vi "AlliGator Load Dataset or Series.vi"(4 "Save Phasor Plot with Overlay":bool, 6 "Save Image with Overlay":bool, 7 "VI in":refnum<vi>, 8 "error in (no error)":errorcluster, 9 "Type of Displayed Image":T1 caption="Displayed Image", 10 "File/Folder Path":path, 11 "AlliGator Ctrl Refnums":T2) -> (0 "error out":errorcluster, 1 "Message":string, 3 "AlliGator Q Elements out":T11[](array[typedef]))   [LabVIEW 2021, in "AlliGator Files.lvlib"]
doc: "Detects type of file loaded and generates the series of actions needed to load it."
uses:
  AlliGator Files.lvlib
  Action Engine/AlliGator Q Element.ctl
  Action Engine/AlliGator Q Event.ctl
  GUI/AlliGator Ctrl Refnums.ctl
  GUI/AlliGator Other Ctrl Refnums.ctl
  GUI/AlliGator State Indicator.ctl
  GUI/AlliGator Main Window Tabs.ctl
  GUI/AlliGator Phasor Plot Ctrl Refnums.ctl
  GUI/AlliGator Phasor Graph Ctrl Refnums.ctl
  Phasor/Phasor Calibration Type.ctl
  GUI/AlliGator Dataset Ctrl Refnums.ctl
  Source Image/AlliGator Displayed Image.ctl
  GUI/AlliGator Registered Events Ctrl Refnums.ctl
  GUI/AlliGator Image Histogram Control Refnums.ctl
  Histograms/Linear Histogram Options.ctl
  Histograms/Histogram Bin Option.ctl
  Histograms/Histogram Bin Position.ctl
  Decay Fit Parameter Map/AlliGator Decay Fit Map Control Refnums.ctl
  Fits/IRF(X)PSED/Decay Fit Parameters & Derived Quantities List v2.ctl
  Parameter Map/AlliGator Parameter Map Control Refnums.ctl
  Files/Load-Save File Info.ctl
  AlliGator FLI Dataset Type.ctl
  ROIs/AlliGator ROI Manager Actions.ctl
  AlliGator Select Folder Mode.ctl
  AlliGator Folder Selection.ctl
  <vilib>/Utility/error.llb/Error Cluster From Error Code.vi
  ROIs/AlliGator Source Image ROI Storage [SGL] v3.vi
  <userlib>/_OpenG.lib/array/array.llb/Filter 1D Array with Scalar (String)__ogtk.vi
  <vilib>/ErrorRing/Error Ring.xnode
  HDF5/AlliGator HDF5.lvlib
  <userlib>/_OpenG.lib/file/file.llb/openg_file.lvlib
  Files/Files.lvlib
  Image/Image.lvlib
  Action Engine/AlliGator Action Engine.lvlib
  <userlib>/_OpenG.lib/array/array.llb/openg_array.lvlib
  ROIs/AlliGator ROIs.lvlib
  Graphs/XY Graph/XY Graph Add-Ons.lvlib
  Globals, Variables, Constants/AlliGator Globals, Variables & Constants.lvlib
  Scripts/AlliGator Scripts.lvlib
  Decay Fit Parameter Map/AlliGator Decay Fit Parameter Map.lvlib
  GUI/GUI.lvlib
  Settings/AlliGator Settings.lvlib
  Sound/Sound.lvlib
  Source Image/AlliGator Source Image.lvlib
  GUI/AlliGator GUI.lvlib
  Phasor/Phasor.lvlib
  Histograms/Histogram Window.lvlib
  Fits/Fits.lvlib
  Parameter Map/AlliGator Parameter Map.lvlib
panel:
  out "Script out":bool
  in  "Script in":bool
  # "see the AlliGator License on the block diagram (Ctrl+E or Window:Show Block Diagram)"
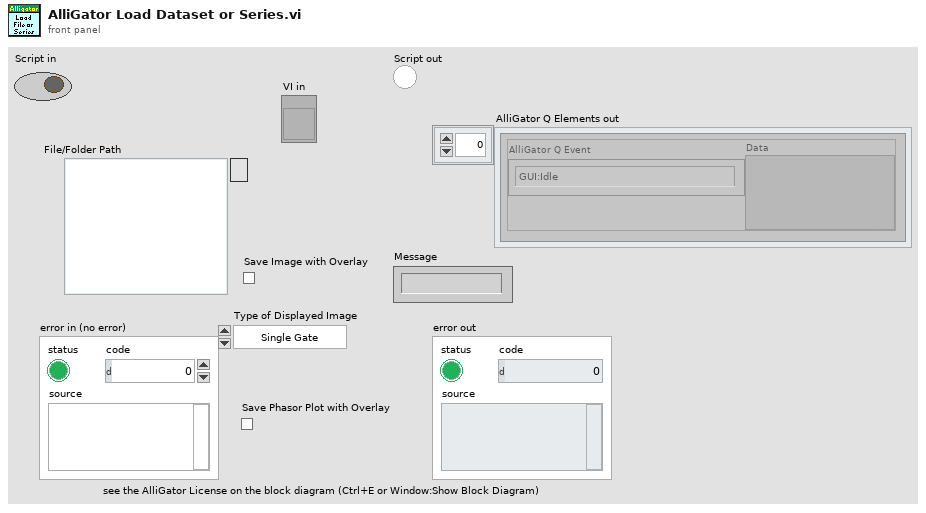
[diagram p1: front panel]
types:
  T1 = typedef "AlliGator Source Image.lvlib/AlliGator Displayed Image.ctl" = enum16{"Single Gate", "Sum of All Gates", "Max of All Gates", "Min of All Gates", "-", "White Ligth Image", "Mask Image"}
  T2 = typedef "AlliGator GUI.lvlib/AlliGator Ctrl Refnums.ctl" = cluster{"Other AlliGator Ctrl Refnums":T3, "Phasor Plot Ctrl Refnums":T4, "Phasor Graph Ctrl Refnums":T5, "Dataset Control References":T6, "Registered Events Ctrl Refnums":T7, "Image Histogram Ctrl Refnums":T8, "Decay Fit Map Ctrl Refums":T9, "Parameter Map Ctrl Refums":T10}
  T3 = typedef "AlliGator GUI.lvlib/AlliGator Other Ctrl Refnums.ctl" = cluster{"State Indicators":refnum<vi>, " Progress Bar":refnum<vi>, "Decay Graph Active":refnum<vi>, "Decay Statistics Bin":refnum<vi>, "Time Step":refnum<vi>, "Use File Timestamp":refnum<vi>, "Tab Control":refnum<vi>, "CPU":refnum<vi>, "Abort Fit":refnum<vi>, "Dataset File/Folder Path":refnum<vi>, "Abort ROI Creation":refnum<vi>, "Event LED":refnum<vi>, "Dataset File/Folder Path 2":refnum<vi>, "Dataset File/Folder Path 3":refnum<vi>, "Dataset File/Folder Path 4":refnum<vi>, "Dataset File/Folder Path 5":refnum<vi>, "Dataset File/Folder Path 6":refnum<vi>, "Dataset File/Folder Path 7":refnum<vi>, "Dataset File/Folder Path 8":refnum<vi>, "Dataset File/Folder Path 9":refnum<vi>, "Dataset File/Folder Path 10":refnum<vi>, "Dataset File/Folder Path 11":refnum<vi>}
  T4 = typedef "AlliGator GUI.lvlib/AlliGator Phasor Plot Ctrl Refnums.ctl" = cluster{"Phasor Ratio":refnum<vi>, "Modulus Lifetime":refnum<vi>, "Phasor at cursor (m, phi)":refnum<vi>, "Phase Lifetime":refnum<vi>, "Phasor at cursor (g, s)":refnum<vi>, "Phasor Plor Average Lifetime":refnum<vi>, "Phasor Plot Active":refnum<vi>, "Save Phasor Plot":refnum<vi>, "Image Overlay Color":refnum<vi>, "Phasor Plot Color Scale":refnum<vi>, "Reference 1 Button":refnum<vi>, "Reference 2 Button":refnum<vi>}
  T5 = typedef "AlliGator GUI.lvlib/AlliGator Phasor Graph Ctrl Refnums.ctl" = cluster{"Phasor Ratio":refnum<vi>, "Modulus Lifetime":refnum<vi>, "Phasor at cursor (m, phi)":refnum<vi>, "Phase Lifetime":refnum<vi>, "Phasor at cursor (g, s)":refnum<vi>, "Phasor Graph Average Lifetime":refnum<vi>, "Phasor Graph Active":refnum<vi>, "Save Phasor Graph":refnum<vi>, "Phasor Frame Slide":refnum<vi>, "Single Step Phasor":refnum<vi>, "Calibration Type":refnum<vi>, "Show Line":refnum<vi>, "Phase Lifetime 1":refnum<vi>, "Phase Lifetime 2":refnum<vi>, "Phasor Graph Frequency":refnum<vi>, "Phasor Reference 1 Control":refnum<vi>, "Phasor Reference 2 Control":refnum<vi>, "Calibration Lifetime":refnum<vi>, "Phase Lifetime SDV":refnum<vi>, "Average Lifetime SDV":refnum<vi>, "Phasor Ratio SDV":refnum<vi>, "Modulus Lifetime SDV":refnum<vi>}
  T6 = typedef "AlliGator GUI.lvlib/AlliGator Dataset Ctrl Refnums.ctl" = cluster{"Current Data":refnum<vi>, "Gate Image Slide":refnum<vi>, "Time Point Slide":refnum<vi>, "Current Time Stamp":refnum<vi>, "Save Image":refnum<vi>, "Displayed Image":refnum<vi>, "Overlay Mode":refnum<vi>, "Phasor Overlay Color":refnum<vi>, "Image Color Scale":refnum<vi>, "Use ROI as Search Area":refnum<vi>, "Source Image ROI Color":refnum<vi>}
  T7 = typedef "AlliGator GUI.lvlib/AlliGator Registered Events Ctrl Refnums.ctl" = cluster{"Time Point Slider":refnum<vi>, "Phasor Plot Display Range":refnum<vi>, "Decay Graph":refnum<vi>, "Decay Statistics Graph":refnum<vi>, "Intensity Time Trace":refnum<vi>, "Phasor Graph":refnum<vi>, "Phasor Ratio Graph":refnum<vi>, "Lifetime Graph":refnum<vi>, "Phasor Plot Display":refnum<vi>, "Source Image Display":refnum<vi>, "Decay Fit Parameter Map Display Range":refnum<vi>, "Decay Fit Parameter Map Display":refnum<vi>, "Parameter Map Display Range":refnum<vi>, "Parameter Map Display":refnum<vi>, "Phasor Plot Display Range":refnum<vi>}
  T8 = typedef "AlliGator GUI.lvlib/AlliGator Image Histogram Control Refnums.ctl" = cluster{"Image Histogram":refnum<vi>, "Image Histogram Options":refnum<vi>, "Image Histogram Active":refnum<vi>, "Image Histogram Upper Percentile":refnum<vi>, "Image Histogram Lower Percentile":refnum<vi>, "Auto-Adjust Contrast":refnum<vi>}
  T9 = typedef "AlliGator Decay Fit Parameter Map.lvlib/AlliGator Decay Fit Map Control Refnums.ctl" = cluster{"Decay Fit Parameter Map Color Scale":refnum<vi>, "Decay Fit Parameter":refnum<vi>, "Max Parameter":refnum<vi>, "Min Parameter":refnum<vi>, "Decay Fit Parameter Map Display":refnum<vi>, "Decay Fit Parameter Map Display Range":refnum<vi>}
  T10 = typedef "AlliGator Parameter Map.lvlib/AlliGator Parameter Map Control Refnums.ctl" = cluster{"Parameter Map Color Scale":refnum<vi>, "Map Parameter":refnum<vi>, "Max Parameter":refnum<vi>, "Min Parameter":refnum<vi>, "Parameter Map Display":refnum<vi>, "Parameter Map Display Range":refnum<vi>, "Parameter Map Set":refnum<vi>}
  T11 = typedef "AlliGator Action Engine.lvlib/AlliGator Q Element.ctl" = cluster{"AlliGator Q Event":T12, "Data":variant}
  T12 = typedef "AlliGator Action Engine.lvlib/AlliGator Q Event.ctl" = enum16{"---- Files ----", "Files:Set Batch Export Files To Save", "Files:Set Dataset Loading & Pre-processing Options", "Files:Check #Frames in Dataset", "Files:Increment Frame Index", "Files:Open Mask Image", "Files:Open White Light Image", "Files:Open Single Dataset", "Files:New Folder of Folders Selected", "Files:Load File (all Types)_Scriptable", "Files:Move Flattened Series to Folders Series", "Files:Select Folder", "Files:Load FLI Dataset", "Files:Load Swiss SPAD 1 Dataset", "Files:Load Swiss SPAD 2 Dataset", "Files:Load .sdt FLI Dataset", "Files:Load .ptu FLI Dataset", "Files:Load .bin FLI Dataset", "Files:Load Single Gate Image Folder", "Files:Load I/m/phi Dataset (deprecated)", "Files:Load Single Image", "Files:Subtract Background File", "Files:Export FLI Dataset", "Files:Load HDF5 FLI Dataset", "Files:Set Destination File Path", "Files:Save Mask Image", "Files:Batch Conversion", "Files:New Folder Selected", "Files:Close FLI Dataset", "Files:Close FLI Dataset Series", "Files:Close White Light Image", "Files:Close Mask Image", "---- FLI Dataset ----", "FLI Dataset:Channel Arithmetic", "FLI Dataset:Export Average Lifetime Map as ASCII", "FLI Dataset:Export User-Defined Quantity Map as ASCII", "FLI Dataset:Python Function FLI Dataset Event", "FLI Dataset:ROI Analysis", "FLI Dataset:Tilted Logistic Square Gated IRF Characteristics Map", "FLI Dataset:Logistic Square Gated IRF Characteristics Map", "FLI Dataset:Square Gated IRF Characteristics Map", "FLI Dataset:Multi-ROI Single-Pixel Phasor Analysis", "FLI Dataset:Multi-ROI Single-Pixel NLSF Analysis", "FLI Dataset:All ROIs IRF Extraction", "FLI Dataset:All ROIs Decay Fit Non-Interactive (Fast + Individual IRF)", "FLI Dataset:All ROIs Phasor Analysis", "FLI Dataset:All ROIs Decay Fit", "FLI Dataset:Fluorescence Decay Statistics", "FLI Dataset:Update Decay Statistics Graph", "FLI Dataset:Get Decay from ROI", "FLI Dataset:All ROIs Average Lifetimes", "FLI Dataset:Save/Load Local IRFs", "FLI Dataset:Clear Local IRFs", "---- FLI Dataset Series ----", "FLI Dataset Series:Sum All Datasets in Series", "FLI Dataset Series:Add Dataset to Accumulated Dataset", "FLI Dataset Series:Display Accumulated Dataset", "FLI Dataset Series:Clear Dataset Series Sum", "FLI Dataset Series:Time-Series Analysis (NLSF)", "FLI Dataset Series:Time-Series Analysis (Phasor)", "---- Image ----", "Image:Update Image Profile Plots", "Image:Image Histogram Cursor Move", "Image:Image Histogram", "Image:Image Contrast", "Image:Set Image Histogram Cursor Move Flag", "Image:Clear Image Overlay", "Image:Use ROI as Search Area", "Image:Set ROI Diameter", "Image:Save Image Data as TIFF", "Image:Save Displayed Image with Overlay", "Image:Save Image Overlay Only", "Image:Save Image as Hot Pixel Mask", "Image:Change Source Image Color Palette", "Image:Copy Image to Clipboard", "Image:Source Image ROI Selection", "Image:Delete All ROIs", "Image:Delete All Unselected ROIs", "Image:Delete ROI", "Image:Merge All ROIs", "Image:Store ROI", "Image:Source Image ROI Storage", "Image:Export ROI Description to Notebook", "Image:Save ROI", "Image:Load ROI", "Image:Paste ROI Definition", "Image:Clear ROI", "Image:Identify ROIs in Mask Image", "Image:Create Complementary ROI", "Image:Create Contour ROI", "Image:Create ROI(s) from Pixels with Peak above Min_Scriptable", "Image:Create ROI(s) from Pixels with Intensity above Min_Scriptable", "Image:Compute ROI Statistics", "Image:Delete ROI(s) based on ROI Characteristics", "Image:Create ROI Grid", "Image:ROI to Individual Pixel ROIs", "Image:Python Function Source Image Event", "Image:Show Phasor Calibration Map ROI Centers", "Image:Convert ROI to Mask Image", "Image:Mouse Move", "Image:Mouse Up", "Image:Set Source Image Mouse Move Flag", "Image:Add Scale Bar Overlay", "Image:Delete Existing ROIs Option", "Image:Overlay ROI Median", "Image:Check Current ROI", "---- Decay ----", "Decay:Clear IRF/Reference Plot", "Decay:Add Decay to Graph", "Decay:Smoothen Plot", "Decay:Smoothen Plot Tail", "Decay:Average Selected Plots", "Decay:Extract IRF", "Decay:Optimal IRF Extraction", "Decay:Threshold IRF", "Decay:Fit to Model IRF", "Decay:Fit IRF to Square Gate", "Decay:Fit IRF to Logistic Square Gate", "Decay:Fit IRF to Tilted Logistic Square Gate", "Decay:Create Bounding Cursors Set", "Decay:Export Bounding Cursors Definition to Notebook", "Decay:Denoise Plot", "Decay:Compute Cumulative Function", "Decay:Use as Reference Decay", "Decay:Show Reference Decay/IRF", "Decay:Extrapolate Decay", "Decay:Create Head & Tail Bounding Cursors", "Decay:Store Cursor-defined Head & Tail Fractions", "Decay:Rebin Plot", "Decay:1-Normalize Decay", "Decay:[0-1]-Normalize Plot", "Decay:Straighten Decay", "Decay:Shift Decay", "Decay:Fold Decay", "Decay:Fit Decay", "Decay:Global Fit of Selected Decays", "Decay:Post Global Fit Script", "Decay:Add Global Fit Parameters to Graph", "Decay:Add Decay Parameter(s) to Plot (Graph)", "Decay:Export Decay to Phasor Graph", "Decay:Plot Decay Shifts", "Decay:Compute Average Lifetime", "Decay:Plot Convolution", "Decay:Graph Tip Strip Update", "---- Decay Statistics ----", "Decay Statistics:Tip Strip Update", "---- Intensity Time Trace ----", "Intensity Time Trace:Use File Timestamp", "Intensity Time Trace:Load Intensity Corrections File", "Intensity Time Trace:Clear Intensity Corrections File", "Intensity Time Trace:Tip Strip Update", "---- Phasor Plot ----", "Phasor Plot:Build Phasor Plot", "Phasor Plot:Change Phasor Plot Color Palette", "Phasor Plot:Adjust Phasor Plot Display Range", "Phasor Plot:Highlight Image ROI in Phasor Plot", "Phasor Plot:Save Phasor Plot Image with Overlay", "Phasor Plot:Export Complex Phasor Map", "Phasor Plot:Export Phasor Ratio Map", "Phasor Plot:Export Average Lifetime Map", "Phasor Plot:Compute Phase Lifetime Histogram", "Phasor Plot:Compute Phasor Ratio Histogram", "Phasor Plot:Compute Phase Lifetime vs Intensity Scatter Plot", "Phasor Plot:Weber 2-Component Decomposition", "Phasor Plot:Update Phasor Color Map Vertices", "Phasor Plot:Clear Phasor Overlay", "Phasor Plot:Use Segment Extremities as References", "Phasor Plot:Use UC/Segment Intersections as References", "Phasor Plot:Use UC/Principal Axis Intersections as References", "Phasor Plot:Use UC/Linear Fit Intersections as References", "Phasor Plot:Update Phasor Plot Reference", "Phasor Plot:Show Local Phasor Info in Phasor Plot", "Phasor Plot:Update Phasor Plot State", "Phasor Plot:Phasor Plot ROI Storage", "Phasor Plot:Phasor Plot ROI Selection", "Phasor Plot:Python Function Phasor Plot Event", "Phasor Plot:Overlay Phasor ROI, Ratio or Map in Source Image", "Phasor Plot:Compute Decay of Selected Phasors", "Phasor Plot:Phasor at Image Pixel", "Phasor Plot:Mouse Move", "Phasor Plot:Mouse Up", "Phasor Plot:Display Range Mouse Move", "Phasor Plot:Set Mouse Move Flag", "---- Phasor Graph ----", "Phasor Graph:Calibrated Phasor Map Series", "Phasor Graph:Whole Image Phasor Scatter Plot (deprecated)", "Phasor Graph:Get Phasor Value", "Phasor Graph:Create New Phasor Plot Dialog", "Phasor Graph:Update Last Phasor Value", "Phasor Graph:Update Phasor (m, phi)", "Phasor Graph:Remove Single Phasor from Plot", "Phasor Graph:Add Single Phasor to Plot", "Phasor Graph:Remove Phasor Plot", "Phasor Graph:Remove Selected Phasor Plots", "Phasor Graph:Clear Phasor Data", "Phasor Graph:Clear Phasor Graph", "Phasor Graph:Cursor Move", "Phasor Graph:Draw Cursor Connecting Line", "Phasor Graph:Clear Cursor Connecting Line", "Phasor Graph:Find UC Intersection", "Phasor Graph:Use UC/Cursor-Defined Line Intersections", "Phasor Graph:Use Selected Plots Fitted Line/UC Intersections", "Phasor Graph:Use Selected Plots Principal Axis/UC Intersections", "Phasor Graph:Show Single Phasor", "Phasor Graph:Save Single Phasor Plot", "Phasor Graph:Save All Phasor Plots", "Phasor Graph:Load Phasor Plot(s)", "Phasor Graph:Phasor Multiplication", "Phasor Graph:Compute Average Phasor", "Phasor Graph:Compute Multiple Average Phasors (Selected Plots)", "Phasor Graph:Export Single Phasor Plot Phase Lifetimes", "Phasor Graph:Phase Lifetime Trajectory (deprecated)", "Phasor Graph:Phase Lifetime vs Intensity Scatter Plot (deprecated)", "Phasor Graph:Parameter 2 vs Parameter 1 Scatter Plot", "Phasor Graph:Use Cursor n Location", "Phasor Graph:Set Reference n to Current Phase Lifetime Value", "Phasor Graph:Set Reference n to Lifetime Value", "Phasor Graph:Set Cursor n Location", "Phasor Graph:Save Phasor Graph Image", "Phasor Graph:Update SEPL Plot", "Phasor Graph:Export Single Phasor Plot Data", "Phasor Graph:Export Selected Phasor Plots Data", "Phasor Graph:Python Function Phasor Graph Event", "Phasor Graph:Tip Strip Update", "---- Calibration ----", "Calibration:Set Calibration Type", "Calibration:Load/Save Phasor Calibration", "Calibration:Load/Save Phasor Calibration Series", "Calibration:Load/Save Phasor Calibration Map", "Calibration:Use as Calibration", "Calibration:Compute Optimal Calibration from Phasor References", "Calibration:Clear Phasor Calibration", "Calibration:Single Phasor Calibration Information", "Calibration:Use as Calibration Series", "Calibration:Use as Calibration Map", "Calibration:Clear Calibration Series", "Calibration:Phasor Calibration Series Information", "Calibration:Clear Calibration Map", "Calibration:Phasor Calibration Map Information", "Calibration:Apply Phasor Calibration", "Calibration:Update Single Plot Calibration", "Calibration:Update Multiple Plots Calibration", "Calibration:Clear Single Plot Calibration", "Calibration:Clear All Plots Calibrations", "Calibration:Clear Plot(s) Calibration(s)?", "Calibration:Phasor Calibration Maps (# Gates Series)", "---- Phasor Ratio ----", "Phasor Ratio:Clear Reference n", "Phasor Ratio:Toggle Selected Plot(s)  Lock to Reference 1", "Phasor Ratio:Use as Reference n", "Phasor Ratio:Send Reference n to Notebook", "Phasor Ratio:Toggle Selected Plot(s)  Lock to Reference 2", "Phasor Ratio:Compute Phasor Ratio at Mouse Location", "Phasor Ratio:Compute Phasor Plot's Average Phasor Ratio", "Phasor Ratio:Compute Time-Series Phasor Ratios", "Phasor Ratio:Fit Line to Phasor Ratio Plot", "Phasor Ratio:Save References", "Phasor Ratio:Load References", "Phasor Ratio:Update Phasor Reference 1", "Phasor Ratio:Update Phasor Reference 2", "Phasor Ratio:Move Cursor n to Reference n", "Phasor Ratio:Use as Phasor Reference 1 Lifetime", "Phasor Ratio:Use as Phasor Reference 2 Lifetime", "Phasor Ratio:Export Phasor Ratio Map as ASCII", "Phasor Ratio:Tip Strip Update", "---- Lifetime & Other Parameters Graph ----", "Lifetime:Power Law from Intensity Distribution", "---- Decay Fit Parameter Map ----", "Decay Fit Parameter Map:Export ROI NLSF Data as ASCII", "Decay Fit Parameter Map:Set Decay Fit Parameter Map Selection", "Decay Fit Parameter Map:Build Decay Fit Parameter Map", "Decay Fit Parameter Map:Change Decay Fit Parameter Map Color Palette", "Decay Fit Parameter Map:Export Decay Fit Parameter Map Data as ASCII", "Decay Fit Parameter Map:Export All Decay Fit Parameter Maps Data as ASCII", "Decay Fit Parameter Map:Selected Parameter Scatterplot", "Decay Fit Parameter Map:Parameter 2 vs Parameter 1 Scatterplot", "Decay Fit Parameter Map:Save Decay Fit Parameter Map Image", "Decay Fit Parameter Map:Save-Load IRFs & Fit Data", "Decay Fit Parameter Map:Update Local Decay Plots", "Decay Fit Parameter Map:Python Function Decay Fit Parameters Map Event", "Decay Fit Parameter Map:Overlay Decay Fit Parameter Map in Source Image", "Decay Fit Parameter Map:Selected Parameter vs Intensity Scatterplot", "Decay Fit Parameter Map:Mouse Up", "Decay Fit Parameter Map:Display Range Mouse Move", "---- Parameter Map ----", "Parameter Map:Export ROI Parameters Data as ASCII", "Parameter Map:Delete Parameter Map Set", "Parameter Map:Update Parameter List", "Parameter Map:Build Parameter Map", "Parameter Map:Change Parameter Map Color Palette", "Parameter Map:Export Parameter Map Data as ASCII", "Parameter Map:Export All Parameter Maps Data as ASCII", "Parameter Map:Selected Parameter Scatterplot", "Parameter Map:Parameter 2 vs Parameter 1 Scatterplot", "Parameter Map:Selected Parameter vs Intensity Scatterplot", "Parameter Map:Save Parameter Map Image", "Parameter Map:Save-Load IRFs & Parameter Maps (TODO)", "Parameter Map:Set Parameter Map Selection", "Parameter Map:Python Function Parameter Map Event", "Parameter Map:Overlay Parameter Map in Source Image", "Parameter Map:Update Local Decay Plots", "Parameter Map:Mouse Up", "Parameter Map:Display Range Mouse Move", "---- Generic Graph ----", "Generic Graph:Generic XY Graph Event", "Generic Graph:Python Function XY Graph Event", "Generic Graph:New Plot", "Generic Graph:Save Plot", "Generic Graph:XY Plot Histogram", "Generic Graph:Set XY Graph Plot Name", "Generic Graph:Set Last Cursor Style", "Generic Graph:Tip Strip Update", "---- GUI ----", "GUI:Start Script", "GUI:Type of Displayed Image Changed", "GUI:Gate Image Slide Changed", "GUI:Show Busy Icon", "GUI:Show Busy Icon & Abort Button", "GUI:Hide Busy Icon", "GUI:Hide Busy Icon & Abort Button", "GUI:Abort", "GUI:End Script", "GUI:Start Timing", "GUI:End Timing", "GUI:Set State Indicator", "GUI:Send Parameters JSON Strings to Clipboard", "GUI:Set Gate Step", "GUI:Idle", "GUI:Initialization", "GUI:Quit", "GUI:Increment Dataset Index", "GUI:Set Dataset Index to -1", "GUI:Time Series Slider Moved", "GUI:Time Series Slider Changed", "GUI:Toggle Playback or Loop", "GUI:Playback Script", "GUI:Set Phasor Frequency", "GUI:Open Window", "GUI:Start Test Script", "GUI:End Test Script", "DEBUG"}
  T13 = typedef "Files.lvlib/Load-Save File Info.ctl" = cluster{"Load/Save":bool, "File Path":path}
  T14 = typedef "AlliGator Files.lvlib/AlliGator FLI Dataset Type.ctl" = enum16{"HDF5 FLI Dataset", "Gate Image Folder", ".sdt FLI Dataset (Becker & Hickl)", ".ptu FLI Dataset (PicoQuant)", "SS1 FLI Dataset", "SS2 FLI Dataset", "I/m/phi Dataset", ".bin FLI Dataset (PicoQuant Binned)", ".bin FLI Dataset (Piccolo Binned)", ".mat FLI Dataset"}
  T15 = typedef "ROI Descriptor" = cluster{"Global Rectangle":i32[], "Contours":cluster{"ID":enum32{"External", "Internal"}, "Type":u32, "Coordinates":i32[]}[]}
  T16 = typedef "AlliGator ROIs.lvlib/AlliGator ROI Manager Actions.ctl" = enum16{"Undefined", "Delete Current ROI", "Delete All Unselected ROIs", "Delete Multiple ROIs", "Delete All ROIs", "Swap ROIs", "Insert ROI", "Update Current ROI Descriptor", "Rename Current ROI", "Store New ROI", "Store Multiple ROIs", "Select Next ROI", "Select Previous ROI", "Find Selected ROI", "Show All ROIs", "Update ROI Manager Window", "Merge All ROIs", "Unmerge ROI", "Set Selected ROI by ID"}
  T17 = typedef "AlliGator Files.lvlib/AlliGator Folder Selection.ctl" = cluster{"Folder Selection Mode":T18, "Folder Path":path}
  T18 = typedef "AlliGator Files.lvlib/AlliGator Select Folder Mode.ctl" = enum16{"Select Gate Folder", "Select Folder of Gate Folders", "Select Folder of SwissSPAD 2 Datasets", "Select Folder of .sdt FLI Datasets (Becker & Hickl)", "Select Folder of .ptu FLI Datasets (PicoQuant)", "Select Folder of .bin FLI Datasets (PicoQuant Binned)", "Select Folder of .bin FLI Datasets (Piccolo Binned)", "Select Folder of HDF5 FLI Datasets"}
  T19 = typedef "AlliGator HDF5 File Type.ctl" = enum16{"FLI Dataset", "Fit Parameter Maps & IRFs", "Local IRFs"}
  T20 = typedef "Image Type" = u32
  T21 = typedef "Fits.lvlib/3-Button Dialog Output.ctl" = enum16{"Window Close", "Button 1", "Button 2", "Button 3"}
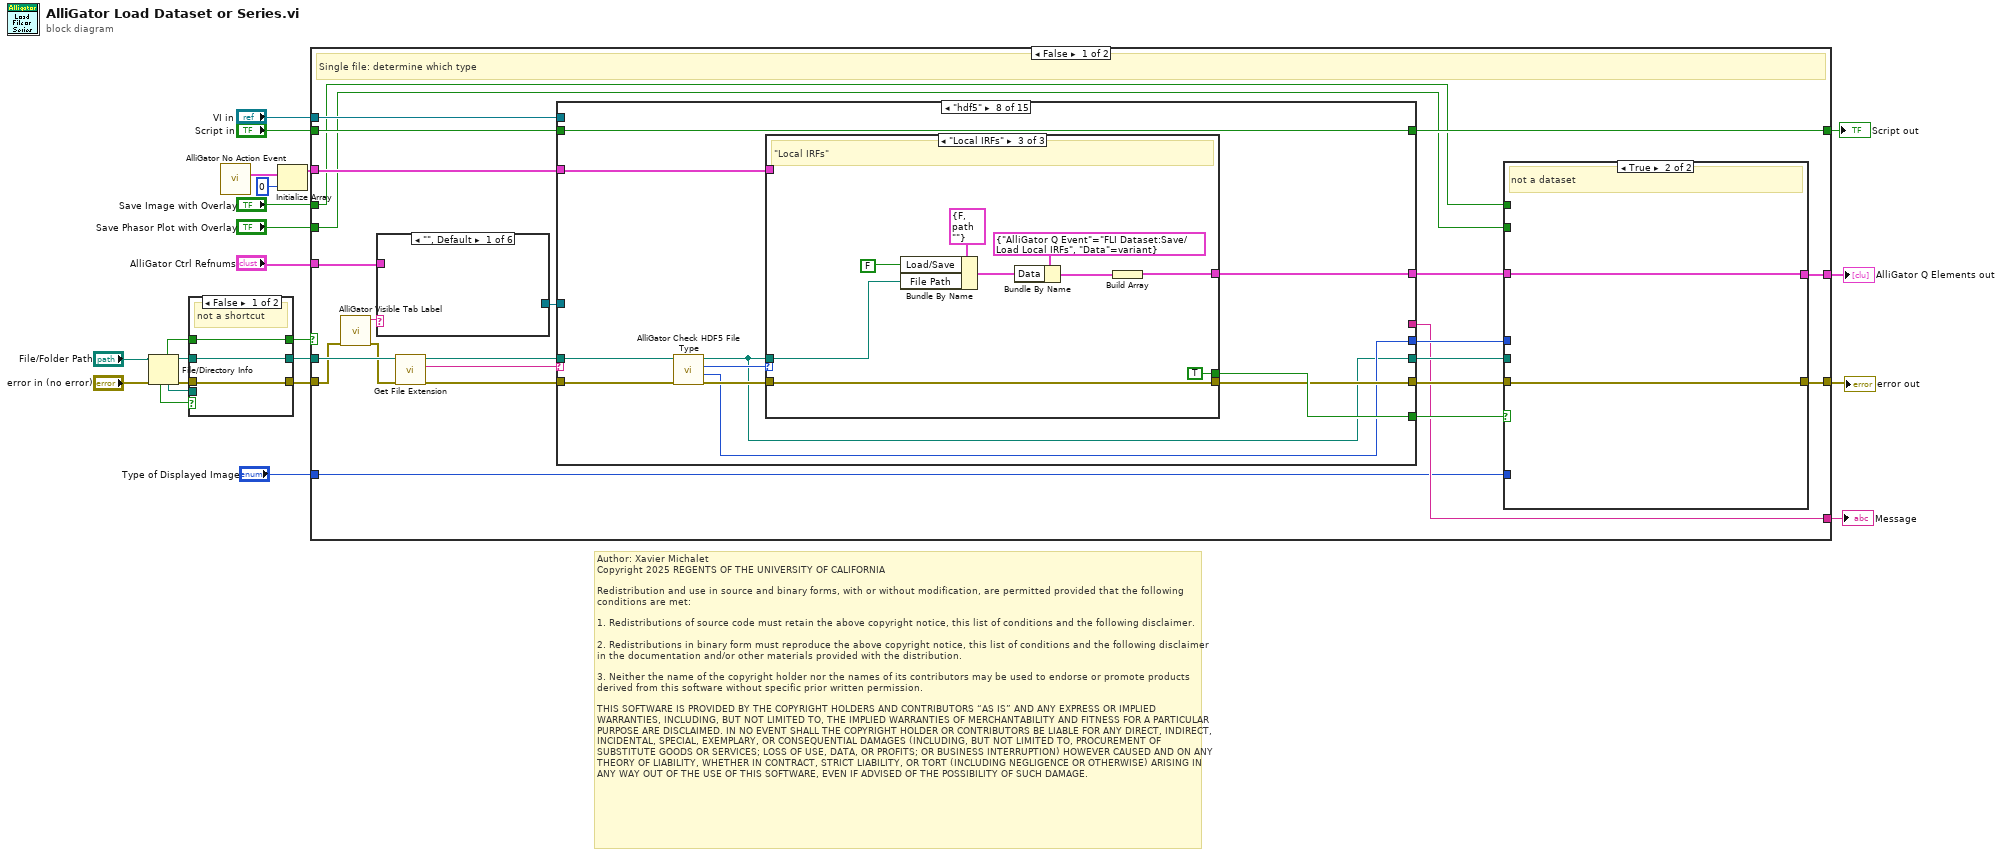
[diagram p0: block diagram]
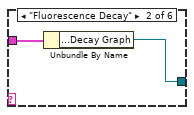
[diagram p2: hidden frame]
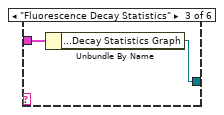
[diagram p3: hidden frame]
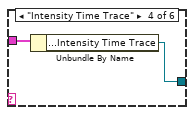
[diagram p4: hidden frame]
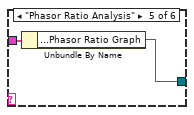
[diagram p5: hidden frame]
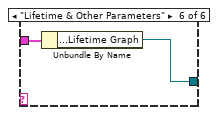
[diagram p6: hidden frame]
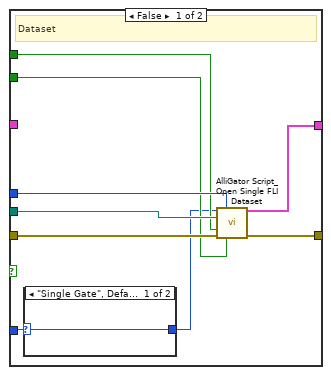
[diagram p7: hidden frame]
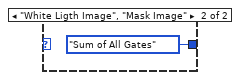
[diagram p8: hidden frame]
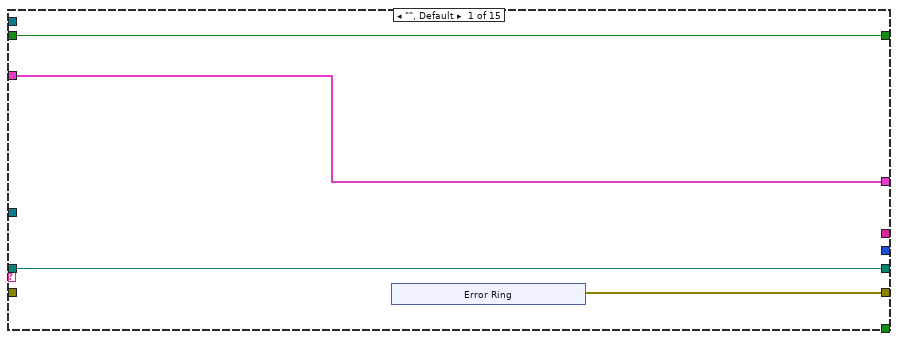
[diagram p9: hidden frame]
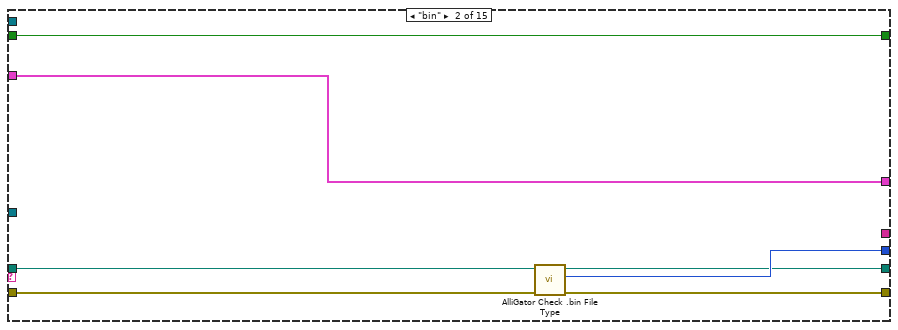
[diagram p10: hidden frame]
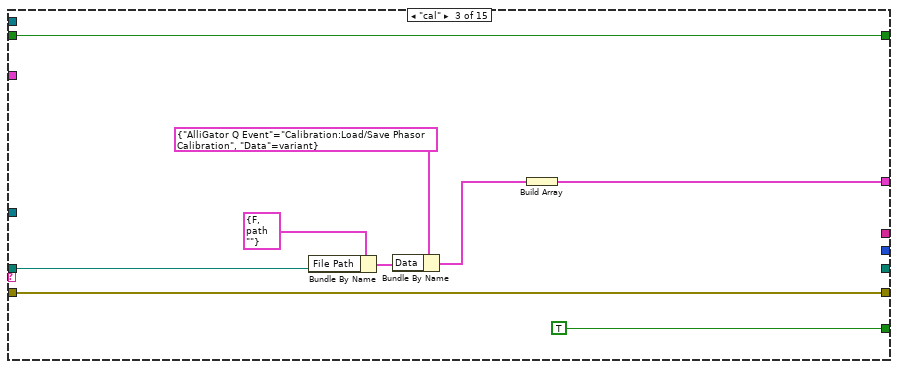
[diagram p11: hidden frame]
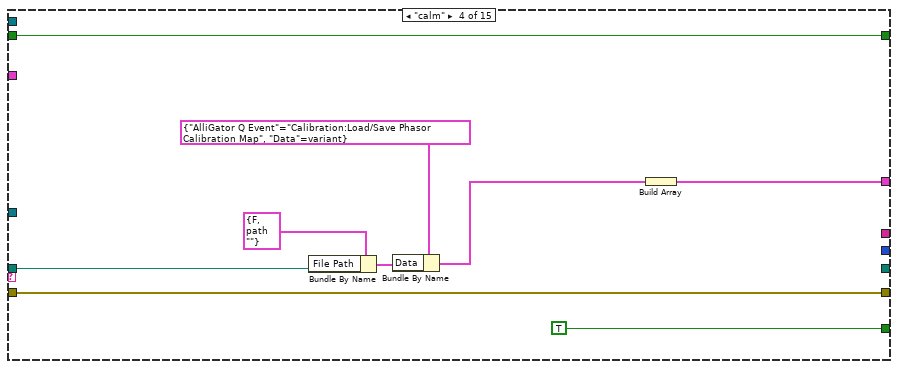
[diagram p12: hidden frame]
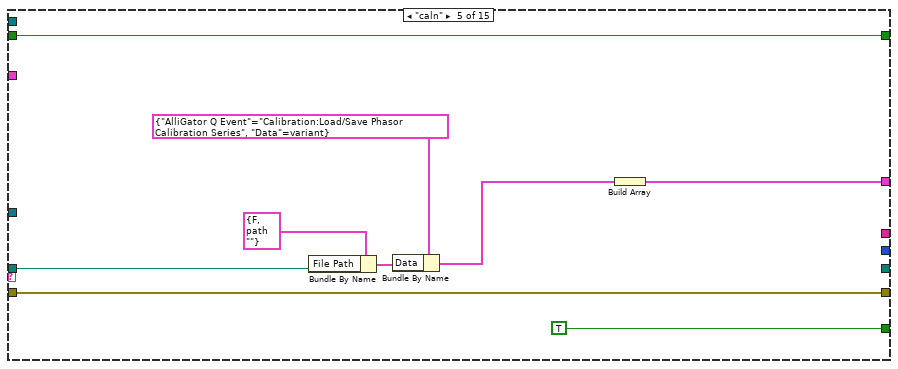
[diagram p13: hidden frame]
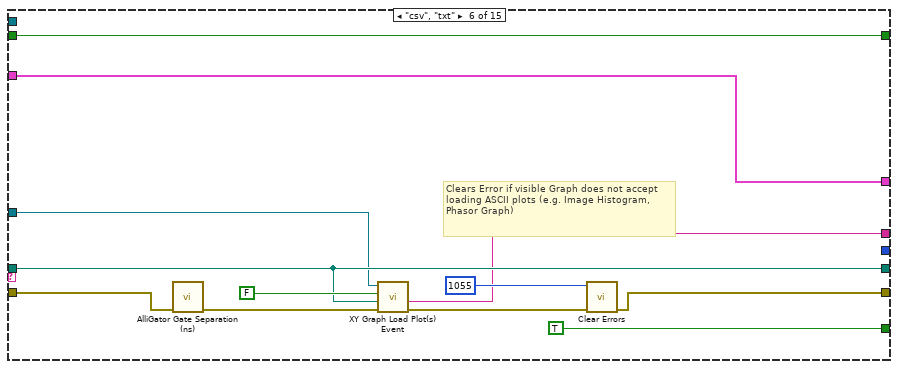
[diagram p14: hidden frame]
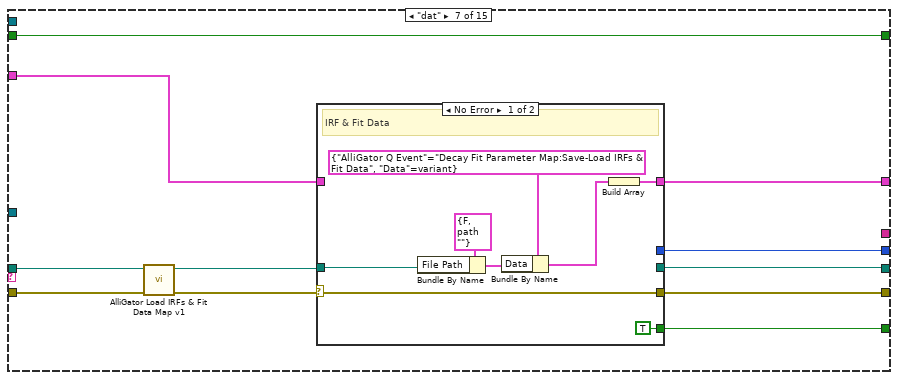
[diagram p15: hidden frame]
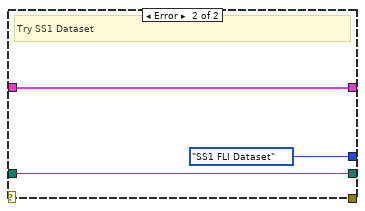
[diagram p16: hidden frame]
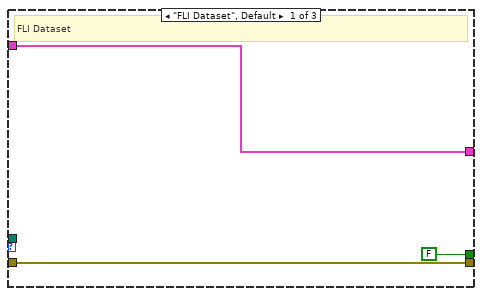
[diagram p17: hidden frame]
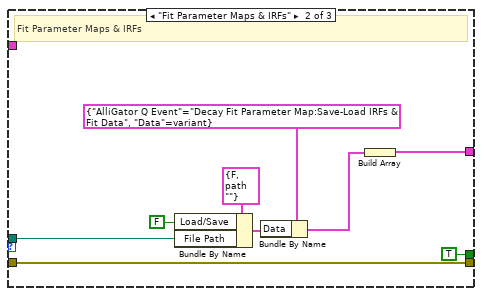
[diagram p18: hidden frame]
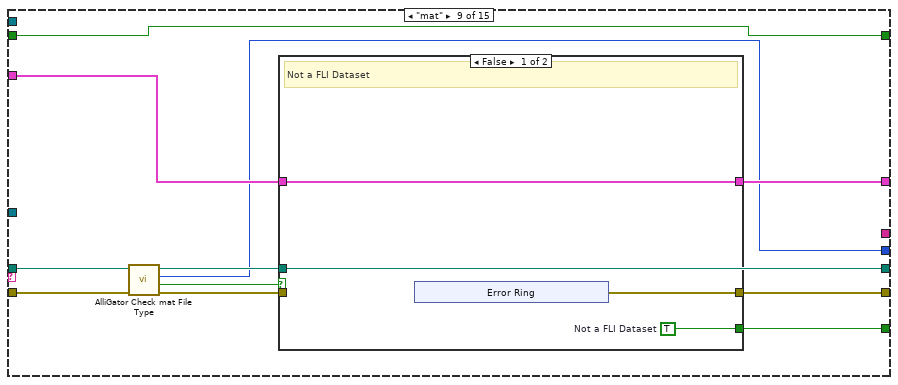
[diagram p19: hidden frame]
diagram:
  # "Author: Xavier Michalet\nCopyright 2025 REGENTS OF THE UNIVERSITY OF CALIFORNIA\n\nRedistribution and use in source and binary forms, with or without modification, are permitted provided that the following conditions are met:\n\n1. Redistributions of source code must retain the above copyright notice, this list of conditions and the following disclaimer.\n\n2. Redistributions in binary form must reproduce the above copyright notice, this list of conditions and the following disclaimer in the documentation and/or other materials provided with the distribution.\n\n3. Neither the name of the copyright holder nor the names of its contributors may be used to endorse or promote products derived from this software without specific prior written permission.\n\nTHIS SOFTWARE IS PROVIDED BY THE COPYRIGHT HOLDERS AND CONTRIBUTORS “AS IS” AND ANY EXPRESS OR IMPLIED WARRANTIES, INCLUDING, BUT NOT LIMITED TO, THE IMPLIED WARRANTIES OF MERCHANTABILITY AND FITNESS FOR A PARTICULAR PURPOSE ARE DISCLAIMED. IN NO EVENT SHALL THE COPYRIGHT HOLDER OR CONTRIBUTORS BE LIABLE FOR ANY DIRECT, INDIRECT, INCIDENTAL, SPECIAL, EXEMPLARY, OR CONSEQUENTIAL DAMAGES (INCLUDING, BUT NOT LIMITED TO, PROCUREMENT OF SUBSTITUTE GOODS OR SERVICES; LOSS OF USE, DATA, OR PROFITS; OR BUSINESS INTERRUPTION) HOWEVER CAUSED AND ON ANY THEORY OF LIABILITY, WHETHER IN CONTRACT, STRICT LIABILITY, OR TORT (INCLUDING NEGLIGENCE OR OTHERWISE) ARISING IN ANY WAY OUT OF THE USE OF THIS SOFTWARE, EVEN IF ADVISED OF THE POSSIBILITY OF SUCH DAMAGE."
  n1 = File/Directory Info(path="File/Folder Path", error in="error in (no error)") -> (path out=w17:path, directory=w14:bool, error out=w16:errorcluster, resolved path=w18:path, shortcut=w19:bool)  [unwired: 2 out]
  n2 = case shown="False" w19 {
    tunnel: w18 -> [_ w31]
    tunnel: w17 -> [w25 _]
    tunnel: w16 -> [w24 w30]
    tunnel: [w26 w29] -> w15
    tunnel: w14 -> [w26 _]
    tunnel: [w25 w28] -> w13
    tunnel: [w24 w27] -> w12
    frame False {
      # "not a shortcut"
    }
    frame True {
      # "Shortcut"
      n3 = File/Directory Info(path=w31, error in=w30) -> (path out=w28:path, directory=w29:bool, error out=w27:errorcluster)  [unwired: 4 out]
    }
  }
  n4 = call "AlliGator No Action Event.vi"() -> ("No Action"=w3:T11)
  n5 = Initialize Array(w3, 0 ("dimension size")) -> (w2:T11[])
  n6 = case shown="False" w15 {
    tunnel: w13 -> [w55 w325]
    tunnel: w12 -> [w46 w324]
    tunnel: [w42 w323] -> w21
    tunnel: [w51 w319] -> w20
    tunnel: "Save Image with Overlay" -> [w33 w316]
    tunnel: "Save Phasor Plot with Overlay" -> [w32 w315]
    tunnel: "AlliGator Ctrl Refnums" -> [w41 _]
    tunnel: w2 -> [w40 _]
    tunnel: [w38 _] -> w8
    tunnel: "VI in" -> [w37 _]
    tunnel: "Script in" -> [w36 w314]
    tunnel: [w35 w314] -> w5
    tunnel: "Type of Displayed Image" -> [w34 w313]
    frame False {
      # "Single file: determine which type"
      n7 = call "AlliGator Visible Tab Label.vi"("Error In"=w46) -> ("Error Out"=w43:errorcluster, "Visible Tab"=w45:string)  [unwired: 9 in]
      n8 = case shown="\"\", Default" w45 {
        tunnel: [_ w56 w58 w60 w62 w64] -> w44
        tunnel: w41 -> [_ w57 w59 w61 w63 w65]
        frame "", Default {
        }
        frame "Fluorescence Decay" {
          n9 = Unbundle By Name(w57) -> ("Registered Events Ctrl Refnums.Decay Graph"=w56:refnum<vi>)
        }
        frame "Fluorescence Decay Statistics" {
          n10 = Unbundle By Name(w59) -> ("Registered Events Ctrl Refnums.Decay Statistics Graph"=w58:refnum<vi>)
        }
        frame "Intensity Time Trace" {
          n11 = Unbundle By Name(w61) -> ("Registered Events Ctrl Refnums.Intensity Time Trace"=w60:refnum<vi>)
        }
        frame "Phasor Ratio Analysis" {
          n12 = Unbundle By Name(w63) -> ("Registered Events Ctrl Refnums.Phasor Ratio Graph"=w62:refnum<vi>)
        }
        frame "Lifetime & Other Parameters" {
          n13 = Unbundle By Name(w65) -> ("Registered Events Ctrl Refnums.Lifetime Graph"=w64:refnum<vi>)
        }
      }
      n14 = call <vilib>:"Get File Extension.vi"("error in (no error)"=w43, "file"=w55) -> ("error out"=w53:errorcluster, "lowercase file extension"=w54:string, "dup file"=w50:path)  [unwired: 5 in, 2 out]
      n15 = case shown="\"hdf5\"" w54 {
        selector: w54 -> [_ _ _ _ _ _ _ _ _ _ _ _ _ w273 _]
        tunnel: w53 -> [_ w89 w97 w105 w114 w125 w139 w164 w196 w214 w249 w258 w263 w272 w311]
        tunnel: [w82 w88 w97 w105 w114 w128 w141 w161 w191 w209 w249 w258 w263 w279 w311] -> w52
        tunnel: [_ w93 _ _ _ _ w143 w156 w187 _ _ AlliGator_FLI_Dataset_Type.".ptu FLI Dataset (PicoQuant)" ("FLI Dataset Type") _ _ AlliGator_FLI_Dataset_Type.".sdt FLI Dataset (Becker & Hickl)" ("FLI Dataset Type")] -> w48
        tunnel: w50 -> [w81 w90 w98 w107 w116 w130 w138 w165 w197 w211 w253 w257 w260 w283 w310]
        tunnel: [w81 w87 _ _ _ w130 w135 w155 w193 _ _ w257 _ w283 w310] -> w49
        tunnel: [_ _ TRUE TRUE TRUE TRUE w140 w163 w194 TRUE TRUE _ TRUE TRUE _] -> w47
        tunnel: w44 -> [_ _ _ _ _ w129 _ _ _ _ _ _ _ _ _]
        tunnel: [w80 w92 w95 w104 w113 w124 w142 w160 w190 w210 w248 w256 w262 w274 w309] -> w39
        tunnel: w40 -> [w80 w92 _ _ _ w124 w134 w159 w189 w208 _ w256 _ w274 w309]
        tunnel: [_ _ _ _ _ w123 _ _ _ _ _ _ _ w269 _] -> w38
        tunnel: w37 -> [_ _ _ _ _ _ _ _ _ _ _ _ _ w278 _]
        tunnel: w36 -> [w79 w91 w94 w103 w112 w121 w133 w158 w188 w207 w247 w255 w261 w275 w308]
        tunnel: [w79 w91 w94 w103 w112 w121 w133 w158 w188 w207 w247 w255 w261 w275 w308] -> w35
        frame "", Default {
          n16 = xnode "Error Ring"() -> ("error out"=w82:errorcluster)
        }
        frame "bin" {
          n17 = call "AlliGator Check .bin File Type.vi"("error in (no error)"=w89, "File Path"=w90) -> ("error out"=w88:errorcluster, "bin FLI Dataset Type"=w93:T14, "File Path dup"=w87:path)  [unwired: 6 in, 1 out]
        }
        frame "cal" {
          n18 = Bundle By Name(cluster=T13 {"Load/Save"=FALSE, "File Path"=path ""}, "File Path"=w98) -> (w99:T13)
          n19 = Bundle By Name(cluster=T11 {"AlliGator Q Event"=enum."Calibration:Load/Save Phasor Calibration", "Data"=variant} ("Alligator Atomic Action"), "Data"=w99) -> (w96:T11)
          n20 = Build Array(w96) -> (w95:T11[])
        }
        frame "calm" {
          n21 = Bundle By Name(cluster=T13 {"Load/Save"=FALSE, "File Path"=path ""}, "File Path"=w107) -> (w108:T13)
          n22 = Bundle By Name(cluster=T11 {"AlliGator Q Event"=enum."Calibration:Load/Save Phasor Calibration Map", "Data"=variant} ("Alligator Atomic Action"), "Data"=w108) -> (w106:T11)
          n23 = Build Array(w106) -> (w104:T11[])
        }
        frame "caln" {
          n24 = Bundle By Name(cluster=T13 {"Load/Save"=FALSE, "File Path"=path ""}, "File Path"=w116) -> (w117:T13)
          n25 = Bundle By Name(cluster=T11 {"AlliGator Q Event"=enum."Calibration:Load/Save Phasor Calibration Series", "Data"=variant} ("Alligator Atomic Action"), "Data"=w117) -> (w115:T11)
          n26 = Build Array(w115) -> (w113:T11[])
        }
        frame "csv", "txt" {
          # "Clears Error if visible Graph does not accept loading ASCII plots (e.g. Image Histogram, Phasor Graph)"
          n27 = call "AlliGator Gate Separation (ns).vi"("error in (no error)"=w125) -> ("error out"=w122:errorcluster)  [unwired: 9 in, 1 out]
          n28 = call "XY Graph Load Plot(s) Event.vi"("Error In"=w122, "File Path"=w130, "Used Dialog? (T)"=FALSE ("Dialog (T)"), "XYGraph Ref"=w129) -> ("Error Out"=w126:errorcluster, "Message"=w123:string)  [unwired: 2 in, 4 out]
          n29 = call <vilib>:"Clear Errors.vi"("error in (no error)"=w126, "specific error code to clear (0: all)"=1055) -> ("error out"=w128:errorcluster)  [unwired: 4 in, 1 out]
        }
        frame "dat" {
          n30 = call "AlliGator Load IRFs & Fit Data Map v1.vi"("error in (no error)"=w139, "File Path in"=w138) -> ("error out"=w136:errorcluster, "File Path out"=w137:path)  [unwired: 7 in, 1 out]
          n31 = case shown="No Error" w136 {
            selector: w136 -> [w145 _]
            tunnel: [_ AlliGator_FLI_Dataset_Type."SS1 FLI Dataset" ("FLI Dataset Type")] -> w143
            tunnel: [w144 w152] -> w142
            tunnel: [w145 _] -> w141
            tunnel: [TRUE _] -> w140
            tunnel: w137 -> [w147 w153]
            tunnel: [_ w153] -> w135
            tunnel: w134 -> [_ w152]
            frame No Error {
              # "IRF & Fit Data"
              n32 = Bundle By Name(cluster=T13 {"Load/Save"=FALSE, "File Path"=path ""}, "File Path"=w147) -> (w151:T13)
              n33 = Bundle By Name(cluster=T11 {"AlliGator Q Event"=enum."Decay Fit Parameter Map:Save-Load IRFs & Fit Data", "Data"=variant} ("Alligator Atomic Action"), "Data"=w151) -> (w146:T11)
              n34 = Build Array(w146) -> (w144:T11[])
            }
            frame Error {
              # "Try SS1 Dataset"
            }
          }
        }
        frame "hdf5" {
          n35 = call "AlliGator Check HDF5 File Type.vi"("error in (no error)"=w164, "HDF5 File Path in"=w165) -> ("error out"=w162:errorcluster, "FLI Dataset Type"=w156:T14, "HDF5 File Type"=w157:T19, "HDF5 File Path out"=w155:path)  [unwired: 6 in]
          n36 = case shown="\"Local IRFs\"" w157 {
            tunnel: [FALSE TRUE TRUE] -> w163
            tunnel: w155 -> [_ w170 w179]
            tunnel: w162 -> [w167 w177 w186]
            tunnel: [w167 w177 w186] -> w161
            tunnel: [w168 w171 w183] -> w160
            tunnel: w159 -> [w168 _ _]
            frame "FLI Dataset", Default {
              # "FLI Dataset"
            }
            frame "Fit Parameter Maps & IRFs" {
              # "Fit Parameter Maps & IRFs"
              n37 = Bundle By Name(cluster=T13 {"Load/Save"=FALSE, "File Path"=path ""} ("Calibration File Information"), "Load/Save"=FALSE, "File Path"=w170) -> (w174:T13)
              n38 = Bundle By Name(cluster=T11 {"AlliGator Q Event"=enum."Decay Fit Parameter Map:Save-Load IRFs & Fit Data", "Data"=variant} ("Alligator Atomic Action"), "Data"=w174) -> (w172:T11)
              n39 = Build Array(w172) -> (w171:T11[])
            }
            frame "Local IRFs" {
              # "\"Local IRFs\""
              n40 = Bundle By Name(cluster=T13 {"Load/Save"=FALSE, "File Path"=path ""} ("Calibration File Information"), "Load/Save"=FALSE, "File Path"=w179) -> (w178:T13)
              n41 = Bundle By Name(cluster=T11 {"AlliGator Q Event"=enum."FLI Dataset:Save/Load Local IRFs", "Data"=variant} ("Alligator Atomic Action"), "Data"=w178) -> (w184:T11)
              n42 = Build Array(w184) -> (w183:T11[])
            }
          }
        }
        frame "mat" {
          n43 = call "AlliGator Check mat File Type.vi"("error in (no error)"=w196, "mat File Path in"=w197) -> ("error out"=w192:errorcluster, "FLI Dataset?"=w195:bool, "FLI Dataset Type"=w187:T14, "mat File Path out"=w193:path)  [unwired: 6 in]
          n44 = case shown="False" w195 {
            tunnel: [w199 _] -> w194
            tunnel: w193 -> [_ _]
            tunnel: w192 -> [_ w206]
            tunnel: [w198 w206] -> w191
            tunnel: [w200 w205] -> w190
            tunnel: w189 -> [w200 w205]
            frame False {
              w199 = TRUE  # Not a FLI Dataset
              # "Not a FLI Dataset"
              n45 = xnode "Error Ring"() -> ("error out"=w198:errorcluster)
            }
            frame True {
              # "FLI Dataset"
            }
          }
        }
        frame "jpeg", "jpg", "png", "tif", "tiff" {
          (unwired) T20 7 items=["Grayscale (U8)", "Grayscale (I16)", "Grayscale (SGL)", "Complex (CSG)", "RGB (U32)", "HSL (U32)", "RGB (U64)", "Grayscale (U16)"] ("Image Type")
          n46 = call "IMAQ GetFileInfo"("error in (no error)"=w214, "File Path"=w211) -> ("error out"=w212:errorcluster, "Image Type"=w213:T20)  [unwired: 3 in, 5 out]
          n47 = case shown="0, 1, 4, 7" w213 {
            tunnel: w212 -> [w217 w227 w246]
            tunnel: w211 -> [_ w225 w245]
            tunnel: [w216 w228 w244] -> w210
            tunnel: [w217 w226 w243] -> w209
            tunnel: w208 -> [w216 w219 _]
            frame 2, Default {
              # "not supported"
              n48 = One Button Dialog(message="Unsupported Image File Format!") -> ()  [unwired: 1 in, 1 out]
              n49 = call "Play Error Sound.vi"() -> ()  [unwired: 27 in, 1 out]
            }
            frame 0, 1, 4, 7 {
              # "U8 or U16: Mask Image or White Light Image"
              n50 = call "Three Buttons Dialog Window.vi"("Window Title"="Single Image Type Selection", "Button 2 Text"="White Light", "Button 1 Text (OK)"="Mask", "Message"="What type of image is this?") -> ("3-button Dialog Output"=w220:T21)  [unwired: 7 in]
              n51 = case shown="\"Button 2\"" w220 {
                tunnel: [w229 w238 w240] -> w228
                tunnel: w227 -> [_ w237 w242]
                tunnel: [w230 w236 w239] -> w226
                tunnel: w225 -> [_ w235 w241]
                tunnel: w219 -> [w229 _ _]
                frame "Window Close", Default {
                  n52 = xnode "Error Ring"() -> ("error out"=w230:errorcluster)
                }
                frame "Button 1" {
                  # "Mask"
                  n53 = call "AlliGator Script Open Mask Image.vi"("Error In"=w237, "Image Path"=w235) -> ("Error Out"=w236:errorcluster, "Action List out"=w238:T11[])  [unwired: 8 in]
                }
                frame "Button 2" {
                  # "White Light"
                  n54 = call "AlliGator Script Open White Light Image.vi"("Error In"=w242, "Image Path"=w241) -> ("Error Out"=w239:errorcluster, "Action List out"=w240:T11[])  [unwired: 8 in]
                }
              }
            }
            frame 16 {
              # "I16 or RGB: white light image"
              n55 = call "AlliGator Script Open White Light Image.vi"("Error In"=w246, "Image Path"=w245) -> ("Error Out"=w243:errorcluster, "Action List out"=w244:T11[])  [unwired: 8 in]
            }
          }
        }
        frame "phplot" {
          n56 = Build Array(w253) -> (w252:path[])
          n57 = Bundle By Name(cluster=T11 {"AlliGator Q Event"=enum."Phasor Graph:Load Phasor Plot(s)", "Data"=variant} ("Alligator Atomic Action"), "Data"=w252) -> (w250:T11)
          n58 = Build Array(w250) -> (w248:T11[])
        }
        frame "ptu" {
        }
        frame "ref" {
          n59 = Bundle By Name(cluster=T11 {"AlliGator Q Event"=enum."Phasor Ratio:Load References", "Data"=variant} ("Alligator Atomic Action"), "Data"=w260) -> (w264:T11)
          n60 = Build Array(w264) -> (w262:T11[])
        }
        frame "roi", "roin" {
          n61 = case shown="\"roi\", Default" w273 {
            tunnel: w272 -> [w288 w292]
            tunnel: [w288 w290] -> w271
            tunnel: [_ w289] -> w268
            frame "roi", Default {
            }
            frame "roin" {
              n62 = call "AlliGator skippable_Delete Existing ROIs Dialog Window.vi"("Error In"=w292) -> ("Error Out"=w291:errorcluster, "Delete"=w293:bool)  [unwired: 9 in]
              n63 = case shown="True" w293 {
                tunnel: w291 -> [w294 w299]
                tunnel: [w294 w297] -> w290
                tunnel: [_ w296] -> w289
                frame False {
                }
                frame True {
                  n64 = call-poly "AlliGator Source Image ROI Storage [PM].vi"("Error In"=w299, "Current ROI Descriptor"=T15 {"Global Rectangle"=[], "Contours"=[]}, "Action"=AlliGator_ROI_Manager_Actions."Delete All ROIs") -> ("Error Out"=w297:errorcluster, "Message"=w296:string)  [unwired: 2 in, 5 out]
                }
              }
            }
          }
          n65 = call "Show Animated Busy Icon with Message.vi"("Already active? (F)"=w275, "Message"="Loading ROI(s)", "Error In"=w271, "Target VI Refnum"=w278) -> ("Error Out"=w280:errorcluster)  [unwired: 7 in]
          n66 = call "AlliGator Load ROI v3.vi"("File Path"=w283, "Error In"=w280, "Destination Image (Source Image)"="Source Image" ("Destination Image"), "Dialog (T)"=FALSE) -> ("Error Out"=w281:errorcluster, "Message"=w276:string, "Phasor Plot Image"=w284:bool)  [unwired: 1 in, 4 out]
          n67 = case shown="True" w284 {
            tunnel: w280 -> [_ w307]
            tunnel: w283 -> [_ w305]
            tunnel: [w301 w303] -> w282
            tunnel: w281 -> [w301 _]
            tunnel: [w300 w302] -> w270
            tunnel: w276 -> [w300 _]
            frame False {
            }
            frame True {
              n68 = call "AlliGator Load ROI v3.vi"("File Path"=w305, "Error In"=w307, "Destination Image (Source Image)"="Phasor Plot Image" ("Destination Image"), "Dialog (T)"=FALSE) -> ("Error Out"=w303:errorcluster, "Message"=w302:string)  [unwired: 1 in, 5 out]
            }
          }
          n69 = Format Into String(format string="\n%s", initial string=w268, w270) -> (resulting string=w269:string)  [unwired: 1 in, 1 out]
          n70 = call "Hide Animated Busy Icon with Message.vi"("Already active? (F)"=w275, "Error In"=w282, "Target VI reference"=w278) -> ("Error Out"=w279:errorcluster)  [unwired: 8 in]
        }
        frame "sdt" {
        }
      }
      n71 = case shown="True" w47 {
        tunnel: w39 -> [_ w78]
        tunnel: w52 -> [w74 w77]
        tunnel: [w73 w77] -> w42
        tunnel: [w72 w78] -> w51
        tunnel: w49 -> [w71 _]
        tunnel: w48 -> [w70 _]
        tunnel: w33 -> [w69 _]
        tunnel: w32 -> [w68 _]
        tunnel: w34 -> [w67 _]
        frame False {
          # "Dataset"
          n72 = case shown="\"Single Gate\", Default" w67 {
            selector: w67 -> [w75 _]
            tunnel: [w75 AlliGator_Displayed_Image."Sum of All Gates" ("Type of Displayed Image")] -> w66
            frame "Single Gate", Default {
            }
            frame "White Ligth Image", "Mask Image" {
            }
          }
          n73 = call "AlliGator Script_Open Single FLI Dataset.vi"("Type of Displayed Image"=w66, "FLI Dataset Type"=w70, "File Path"=w71, "Save Image with Overlay"=w69, "Error In"=w74, "Save Phasor Plot with Overlay"=w68) -> ("Action List out"=w72:T11[], "Error Out"=w73:errorcluster)  [unwired: 8 in]
        }
        frame True {
          # "not a dataset"
        }
      }
    }
    frame True {
      # "Folder: is it a Gate Folder or a Series?"
      n74 = call <userlib>:"List Directory__ogtk.vi"("error in (no error)"=w324, "directory path"=w325) -> ("error out"=w320:errorcluster, "directory names"=w318:string[], "file names"=w317:string[], "dup directory path"=w321:path)  [unwired: 2 in]
      n75 = Empty Array?(array=w317) -> (empty?=w322:bool)
      n76 = case shown="False" w322 {
        tunnel: w321 -> [w339 w438]
        tunnel: w320 -> [w338 w437]
        tunnel: [w335 w440] -> w323
        tunnel: [w334 w439] -> w319
        tunnel: w318 -> [w328 w442]
        tunnel: w317 -> [w331 _]
        tunnel: w316 -> [w330 w436]
        tunnel: w315 -> [w329 w435]
        tunnel: w313 -> [w326 _]
        frame False {
          # "files are present: are they gate images?"
          n77 = Empty Array?(array=w328) -> (empty?=w327:bool)
          n78 = call "Vision Toolkit Supported Files.vi"() -> ("Pattern String"=w340:string)  [unwired: 7 in, 1 out]
          n79 = call "Get Ordered List of Files.vi"("pattern"=w340, "Split string"="_Delay=", "Error In"=w338, "Folder Path"=w339) -> ("Error Out"=w336:errorcluster, "Folder Path dup"=w333:path, "Ordered File Paths"=w332:path[])  [unwired: 4 in, 1 out]
          n80 = Empty Array?(array=w332) -> (empty?=w337:bool)
          n81 = case shown="True" w337 {
            tunnel: w336 -> [w350 w359]
            tunnel: [w346 w360] -> w335
            tunnel: [w344 w358] -> w334
            tunnel: w333 -> [w345 w357]
            tunnel: w331 -> [_ w353]
            tunnel: w330 -> [w349 w356]
            tunnel: w329 -> [w348 w355]
            tunnel: w327 -> [_ w354]
            tunnel: w326 -> [w343 _]
            frame False {
              # "Images found: go for single gate image folder"
              n82 = case shown="\"White Ligth Image\", \"Mask Image\"" w343 {
                selector: w343 -> [w351 _]
                tunnel: [w351 AlliGator_Displayed_Image."Sum of All Gates" ("Type of Displayed Image")] -> w342
                frame "Single Gate", Default {
                }
                frame "White Ligth Image", "Mask Image" {
                }
              }
              n83 = call "AlliGator Script_Open Single FLI Dataset.vi"("Type of Displayed Image"=w342, "FLI Dataset Type"=AlliGator_FLI_Dataset_Type."Gate Image Folder", "File Path"=w345, "Save Image with Overlay"=w349, "Error In"=w350, "Save Phasor Plot with Overlay"=w348) -> ("Action List out"=w344:T11[], "Error Out"=w346:errorcluster)  [unwired: 8 in]
            }
            frame True {
              w362 = string[] ["hdf5", "sdt", "ptu", "bin", "dat"] ("pattern")
              (unwired) "*.hdf5;*.sdt;*.ptu;*.bin;;*.dat" ("pattern")
              # "not gate images: try valid datasets"
              n84 = for {
                tunnel: w353 -> [w434] mode=indexing
                tunnel: [w432] -> w365 mode=indexing
                n85 = String To Path(string=w434) -> (path=w433:path)
                n86 = call <vilib>:"Get File Extension.vi"("file"=w433) -> ("lowercase file extension"=w432:string)  [unwired: 6 in, 4 out]
              }
              n87 = for {
                shift-right: [w429] -> _
                shift-left: w365 -> [w431]
                tunnel: w362 -> [w430] mode=indexing
                tunnel: [w427] -> w364 mode=indexing
                n88 = call-poly <userlib>:"Filter 1D Array__ogtk.vi"("items to filter"=w430, "array"=w431) -> ("filtered item indices"=w428:i32[], "filtered array"=w429:string[])  [unwired: 4 in]
                n89 = Array Size(array=w428) -> (size(s)=w427:i32)
              }
              n90 = Array Max & Min(array=w364) -> (max value=w361:i32, max index (indices)=w363:i32)  [unwired: 2 out]
              n91 = case shown="0" w361 {
                tunnel: w363 -> [_ w408]
                tunnel: w362 -> [_ w407]
                tunnel: [w368 w393] -> w360
                tunnel: w359 -> [w371 w400]
                tunnel: [w372 w394] -> w358
                tunnel: w357 -> [w367 w392]
                tunnel: w356 -> [w370 w398]
                tunnel: w355 -> [w369 w397]
                tunnel: w354 -> [w366 _]
                tunnel: w353 -> [_ w391]
                frame 0 {
                  # "No valid file"
                  n92 = case shown="False" w366 {
                    tunnel: [w373 w386] -> w368
                    tunnel: [w374 _] -> w372
                    tunnel: w367 -> [w381 _]
                    tunnel: w371 -> [w379 _]
                    tunnel: w370 -> [w378 _]
                    tunnel: w369 -> [w377 _]
                    frame False {
                      # "subfolders are present: try folder of gate image folders"
                      n93 = Bundle(cluster=T17 {"Folder Selection Mode"=enum."Select Gate Folder", "Folder Path"=path ""} ("Folder Selection"), "Folder Selection Mode"=AlliGator_Select_Folder_Mode."Select Folder of Gate Folders", "Folder Path"=w381) -> (w383:T17)
                      n94 = Bundle By Name(cluster=T11 {"AlliGator Q Event"=enum."Files:Select Folder", "Data"=variant} ("Time-Gated Phasor Q Element"), "Data"=w383) -> (w380:T11)
                      n95 = call "AlliGator Post Loading Action List.vi"("Error In"=w379, "Save Phasor Plot with Overlay (F)"=w377, "Save Image with Overlay (F)"=w378, "Load Image only? (F)"=FALSE ("Load Image only?")) -> ("Error Out"=w373:errorcluster, "Action List"=w375:T11[])  [unwired: 6 in]
                      n96 = Build Array (concatenate)(w380, w375) -> (w374:T11[])
                    }
                    frame True {
                      # "No subfolders: invalid selection"
                      n97 = xnode "Error Ring"() -> ("error out"=w386:errorcluster)
                    }
                  }
                }
                frame 1, Default {
                  # "looks for the majority type"
                  n98 = Index Array(array=w407, index=w408) -> (element=w401:string)
                  n99 = case shown="\"bin\"" w401 {
                    tunnel: [_ AlliGator_Select_Folder_Mode."Select Folder of HDF5 FLI Datasets" AlliGator_Select_Folder_Mode."Select Folder of .sdt FLI Datasets (Becker & Hickl)" AlliGator_Select_Folder_Mode."Select Folder of .ptu FLI Datasets (PicoQuant)" w420] -> w405
                    tunnel: w400 -> [_ w414 w416 w418 w422]
                    tunnel: [w409 w414 w416 w418 w421] -> w399
                    tunnel: w392 -> [_ _ _ _ w425]
                    tunnel: w391 -> [_ _ _ _ w426]
                    frame "", Default {
                      n100 = xnode "Error Ring"() -> ("error out"=w409:errorcluster)
                    }
                    frame "hdf5" {
                    }
                    frame "sdt" {
                    }
                    frame "ptu" {
                    }
                    frame "bin" {
                      n101 = Index Array(array=w426) -> (element=w424:string)  [unwired: 1 in]
                      n102 = Build Path(base path=w425, name or relative path=w424) -> (appended path=w423:path)
                      n103 = call "AlliGator Check .bin File Type.vi"("error in (no error)"=w422, "File Path"=w423) -> ("error out"=w421:errorcluster, "Folder Selection Mode"=w420:T18)  [unwired: 6 in, 2 out]
                    }
                  }
                  n104 = Bundle(cluster=T17 {"Folder Selection Mode"=enum."Select Gate Folder", "Folder Path"=path ""} ("Folder Selection"), "Folder Selection Mode"=w405, "Folder Path"=w392) -> (w404:T17)
                  n105 = call "AlliGator Post Loading Action List.vi"("Error In"=w399, "Save Phasor Plot with Overlay (F)"=w397, "Save Image with Overlay (F)"=w398, "Load Image only? (F)"=FALSE ("Load Image only?")) -> ("Error Out"=w393:errorcluster, "Action List"=w396:T11[])  [unwired: 6 in]
                  n106 = Bundle By Name(cluster=T11 {"AlliGator Q Event"=enum."Files:Select Folder", "Data"=variant} ("Time-Gated Phasor Q Element"), "Data"=w404) -> (w402:T11)
                  n107 = Build Array (concatenate)(w402, w396) -> (w394:T11[])
                }
              }
            }
          }
        }
        frame True {
          # "No valid file: try folder of gate image folders"
          n108 = Empty Array?(array=w442) -> (empty?=w441:bool)
          n109 = case shown="False" w441 {
            tunnel: [w443 w456] -> w440
            tunnel: [w444 _] -> w439
            tunnel: w438 -> [w451 _]
            tunnel: w437 -> [w449 _]
            tunnel: w436 -> [w448 _]
            tunnel: w435 -> [w447 _]
            frame False {
              # "subfolders are present: try folder of gate image folders"
              n110 = Bundle(cluster=T17 {"Folder Selection Mode"=enum."Select Gate Folder", "Folder Path"=path ""} ("Folder Selection"), "Folder Selection Mode"=AlliGator_Select_Folder_Mode."Select Folder of Gate Folders", "Folder Path"=w451) -> (w453:T17)
              n111 = Bundle By Name(cluster=T11 {"AlliGator Q Event"=enum."Files:Select Folder", "Data"=variant} ("Time-Gated Phasor Q Element"), "Data"=w453) -> (w450:T11)
              n112 = call "AlliGator Post Loading Action List.vi"("Error In"=w449, "Save Phasor Plot with Overlay (F)"=w447, "Save Image with Overlay (F)"=w448, "Load Image only? (F)"=FALSE ("Load Image only?")) -> ("Error Out"=w443:errorcluster, "Action List"=w445:T11[])  [unwired: 6 in]
              n113 = Build Array (concatenate)(w450, w445) -> (w444:T11[])
            }
            frame True {
              # "No subfolders: invalid selection"
              n114 = xnode "Error Ring"() -> ("error out"=w456:errorcluster)
            }
          }
        }
      }
    }
  }
  "AlliGator Q Elements out" <- w20
  "error out" <- w21
  "Message" <- w8
  "Script out" <- w5
